vi "生成word报表.vi"(0 "Array输入":refnum<vi>, 1 "产品序号":string, 2 "标注图":T1(plugin-control), 3 "Array输入 2":refnum<vi>, 4 "测试人":string, 5 "部位":string, 6 "ROI左上角X":i32, 7 "ROI左上角Y":i32, 8 "反射图":T1(plugin-control) caption="Original Image", 9 "框号":dbl format="%#_13g") -> (14 "报告生成路径":path)   [LabVIEW 2018]
uses:
  <vilib>/Utility/NIReport.llb/Report Type.ctl
  <vilib>/Utility/NIReport.llb/Append Report Text (str wrap).vi
  <vilib>/addons/_office/word.llb/Word Edit Cell ([dbl]).vi
  <vilib>/addons/_office/word.llb/Word Edit Cell (str).vi
  <vilib>/Utility/NIReport.llb/Append Report Text (num wrap).vi
  <vilib>/Utility/NIReport.llb/NI_report.lvclass
  <vilib>/addons/_office/NI_ReportGenerationToolkit.lvlib
  <vilib>/Utility/NIReport.llb/Word/NI_Word.lvclass
  <vilib>/Utility/NIReport.llb/NI_ReportGenerationCore.lvlib
  <vilib>/addons/_office/word.llb/Word Edit Cell ([str]).vi
panel:
  out "绝对位置Y2":dbl[](array[numeric])
  out "绝对位置X2":dbl[](array[numeric])
  out "绝对位置Y":dbl[](array[numeric])
  out "绝对位置X":dbl[](array[numeric])
  out "分层累计缺陷占比":dbl
  out "分层Z值":dbl[](array[numeric])
  out "缺陷个数 2":i32
  out "分层数据":dbl[][](array[numeric])
  out "弥散累计缺陷占比":dbl
  out "弥散数据":dbl[][](array[numeric])
  out "弥散Z值":dbl[](array[numeric])
  out "缺陷个数":i32
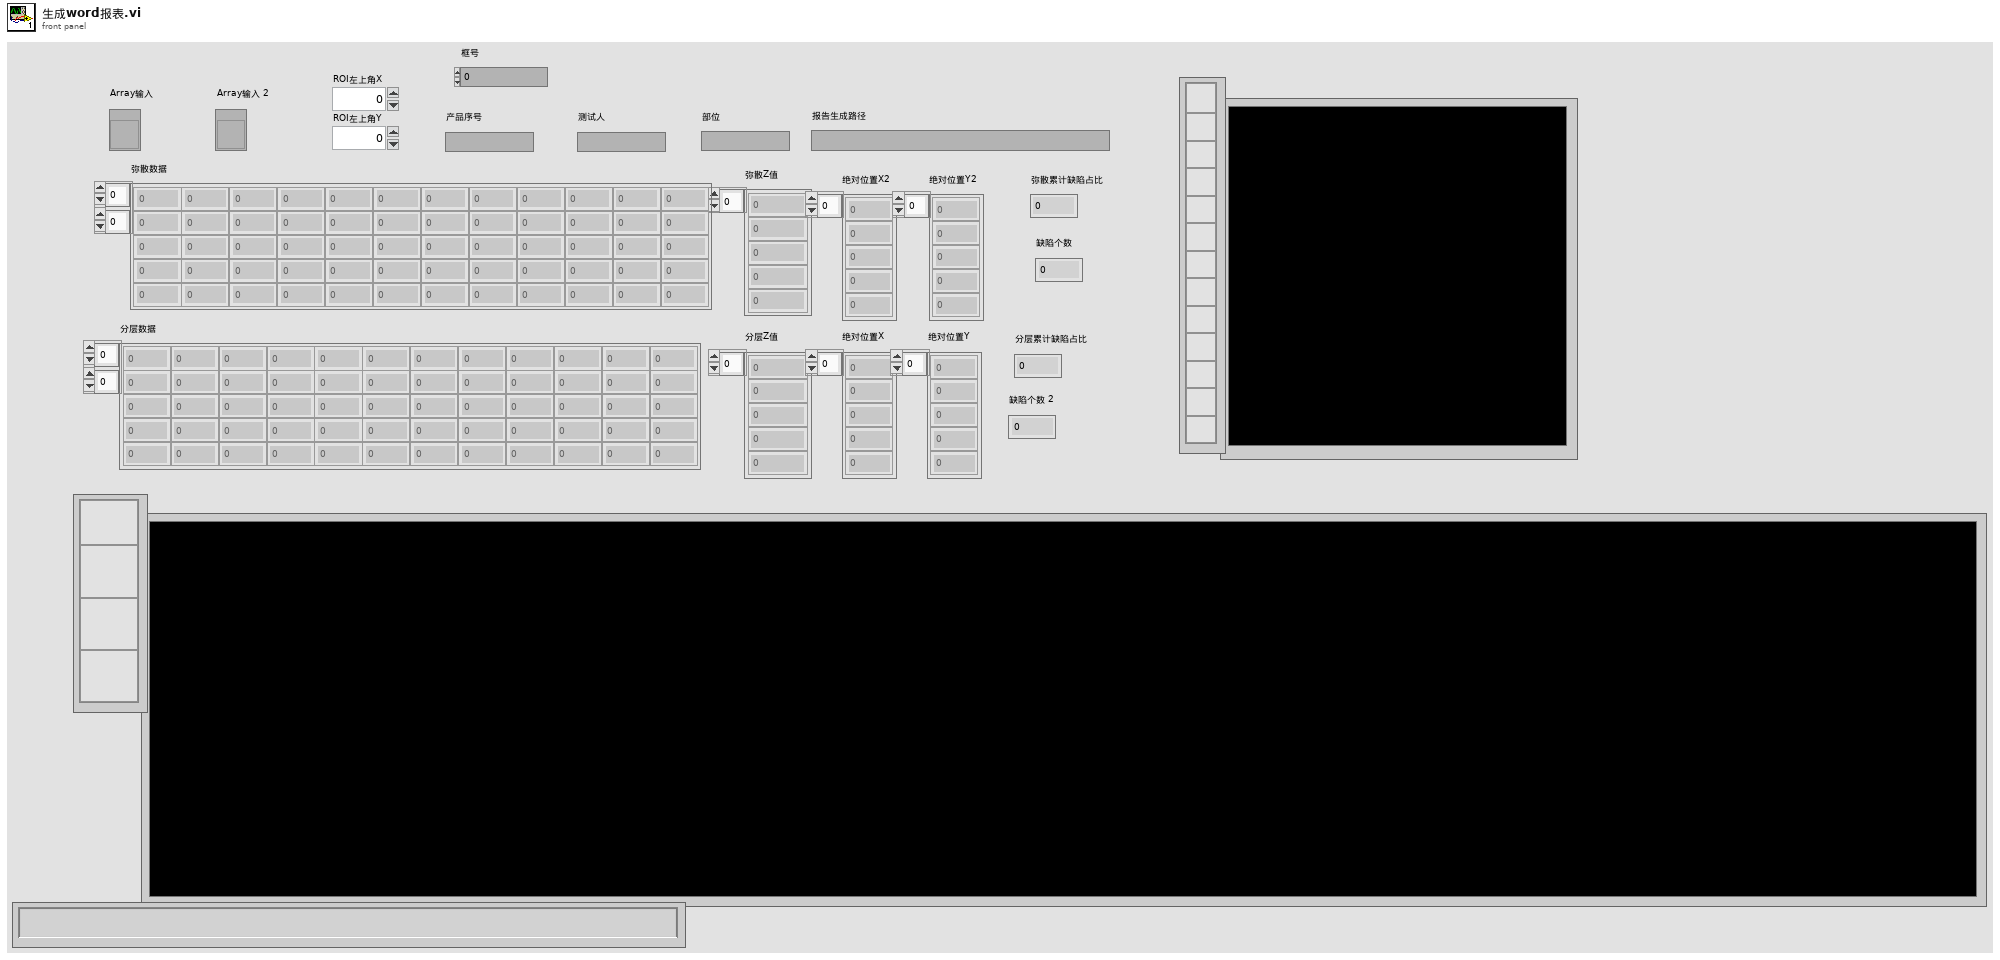
[diagram p1: front panel]
types:
  T1 = typedef "IMAQ Image.ctl" = refnum<image>
  T2 = cluster{"position (Excel)":cluster{"row":i32, "column":i32}, "name (Excel)":string, "bookmark (Word)":string}
  T3 = typedef "NI_ReportGenerationCore.lvlib/Report Type.ctl" = enum16{"HTML", "Word", "Excel"}
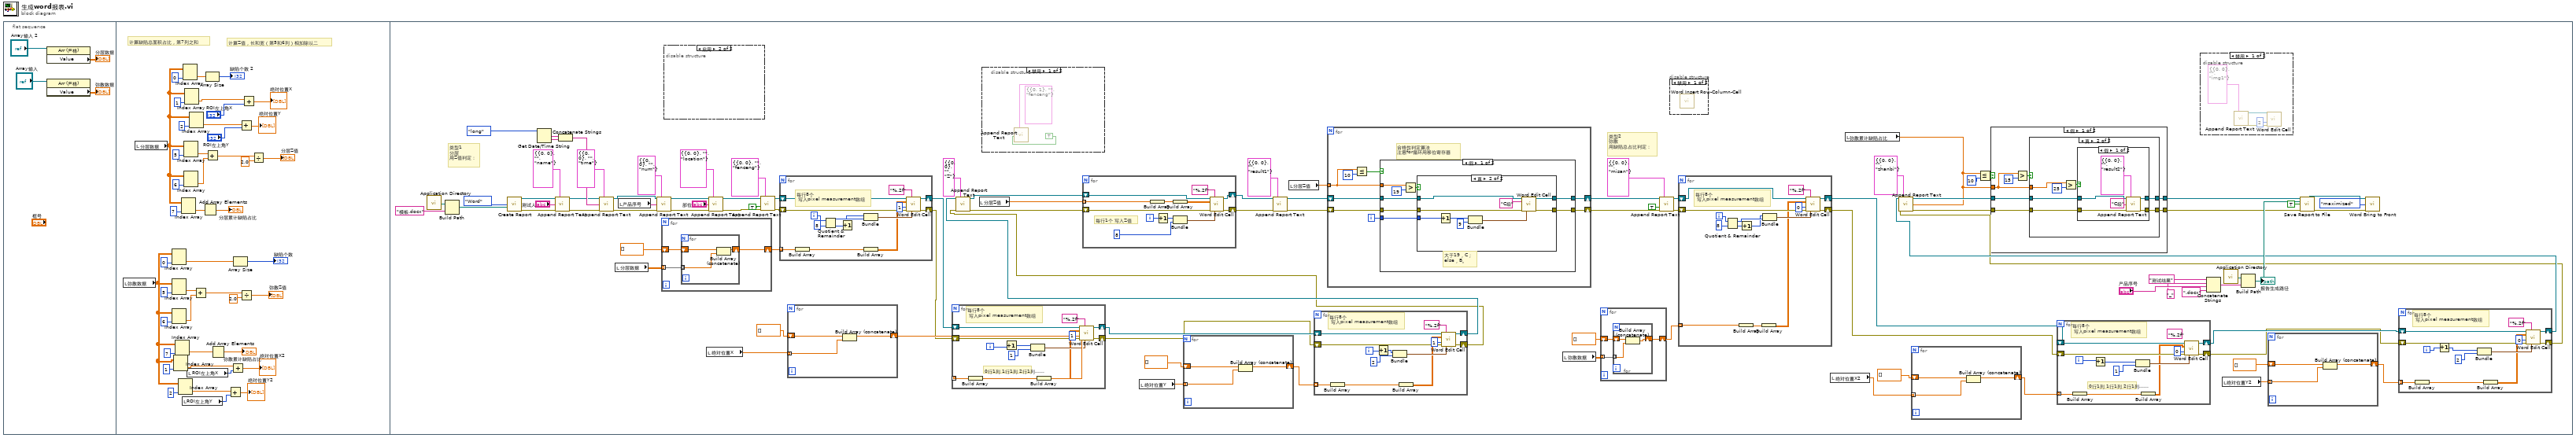
[diagram p0: block diagram]
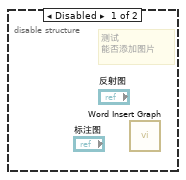
[diagram p5: hidden frame]
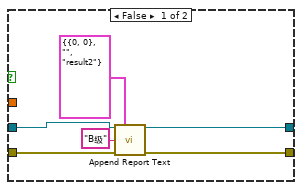
[diagram p6: hidden frame]
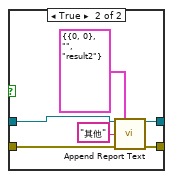
[diagram p7: hidden frame]
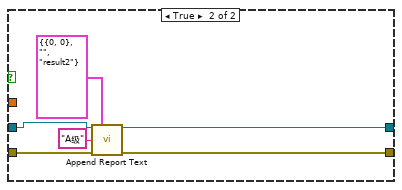
[diagram p8: hidden frame]
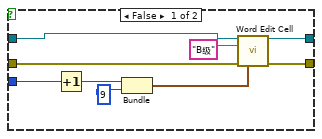
[diagram p9: hidden frame]
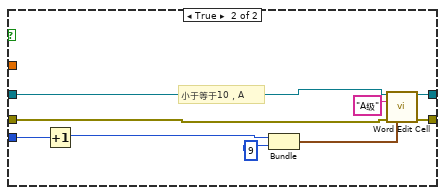
[diagram p10: hidden frame]
diagram:
  n1 = flat-sequence {
    frame #0 {
      n2 = property class="Arr (严格)"(reference="Array输入 2") -> ("Value"=→"分层数据":dbl[][])  [unwired: 1 in, 2 out]
      n3 = property class="Arr (严格)"(reference="Array输入") -> ("Value"=→"弥散数据":dbl[][])  [unwired: 1 in, 2 out]
    }
    frame #1 {
      # "计算缺陷总面积占比，第7列之和"
      # "计算Z值，长和宽（第5和6列）相加除以二"
      n4 = local read "弥散数据"() -> (w7:dbl[][])
      n5 = local read "分层数据"() -> (w20:dbl[][])
      n6 = Index Array(array=w7, index (col)=0 ("禁用的索引 (列)")) -> (element=w46:dbl[])  [unwired: 1 in]
      n7 = Index Array(array=w7, index (col)=5 ("索引")) -> (element=w43:dbl[])  [unwired: 1 in]
      n8 = Index Array(array=w7, index (col)=6 ("索引")) -> (element=w44:dbl[])  [unwired: 1 in]
      n9 = Index Array(array=w7, index (col)=1 ("索引 (列)")) -> (element=w11:dbl[])  [unwired: 1 in]
      n10 = Index Array(array=w7, index (col)=7 ("禁用的索引 (列)")) -> (element=w37:dbl[])  [unwired: 1 in]
      n11 = Index Array(array=w7, index (col)=2 ("索引 (列)")) -> (element=w9:dbl[])  [unwired: 1 in]
      n12 = Index Array(array=w20, index (col)=7 ("禁用的索引 (列)")) -> (element=w24:dbl[])  [unwired: 1 in]
      n13 = local read "ROI左上角Y"() -> (w5:i32)
      n14 = Index Array(array=w20, index (col)=0 ("禁用的索引 (列)")) -> (element=w33:dbl[])  [unwired: 1 in]
      n15 = Index Array(array=w20, index (col)=5 ("索引")) -> (element=w30:dbl[])  [unwired: 1 in]
      n16 = Index Array(array=w20, index (col)=6 ("索引")) -> (element=w31:dbl[])  [unwired: 1 in]
      n17 = Index Array(array=w20, index (col)=1 ("索引 (列)")) -> (element=w19:dbl[])  [unwired: 1 in]
      n18 = local read "ROI左上角X"() -> (w6:i32)
      n19 = Index Array(array=w20, index (col)=2 ("索引 (列)")) -> (element=w16:dbl[])  [unwired: 1 in]
      n20 = Add(x=w43, y=w44) -> (x+y=w45:dbl[])
      n21 = Add Array Elements(numeric array=w24) -> (sum=→"分层累计缺陷占比":dbl)
      n22 = Array Size(array=w33) -> (size(s)=→"缺陷个数 2":i32)
      n23 = Add(x=w30, y=w31) -> (x+y=w32:dbl[])
      n24 = Add Array Elements(numeric array=w37) -> (sum=→"弥散累计缺陷占比":dbl)
      n25 = Add(x=w9, y=w5) -> (x+y=→"绝对位置Y2":dbl[])
      n26 = Add(x=w11, y=w6) -> (x+y=→"绝对位置X2":dbl[])
      n27 = Array Size(array=w46) -> (size(s)=→"缺陷个数":i32)
      n28 = Add(x=w16, y="ROI左上角Y") -> (x+y=→"绝对位置Y":dbl[])
      n29 = Divide(x=w45, y=2.0) -> (x/y=→"弥散Z值":dbl[])
      n30 = Add(x=w19, y="ROI左上角X") -> (x+y=→"绝对位置X":dbl[])
      n31 = Divide(x=w32, y=2.0) -> (x/y=→"分层Z值":dbl[])
    }
    frame #2 {
      # "类型2\n弥散\n用缺陷总占比判定："
      # "类型1\n分层\n用Z值判定："
      n32 = call <vilib>:"Application Directory.vi"() -> ("Application Directory"=w125:path)
      n33 = Build Path(base path=w125, name or relative path="模板.docx") -> (appended path=w124:path)
      n34 = call <vilib>:"Create Report.vi"("report type"=Report_Type."Word" ("Report Type"), "template (empty)"=w124) -> ("report out"=w117:refnum<class "NI_report.lvclass">, "error out"=w114:errorcluster)  [unwired: 12 in]
      n35 = Get Date/Time String(date format (0)=enum16{"short", "long", "abbreviated"}."long" ("日期格式(0)")) -> (date string=w123:string, time string=w121:string)  [unwired: 2 in]
      n36 = call-poly <vilib>:"Append Report Text.vi"("report in"=w117, "MS Office parameters"=T2 {"position (Excel)"={"row"=0, "column"=0}, "name (Excel)"="", "bookmark (Word)"="name"}, "text"="测试人", "error in (no error)"=w114) -> ("report out"=w116:refnum<class "NI_report.lvclass">, "error out"=w115:errorcluster)  [unwired: 8 in, 2 out]
      n37 = Concatenate Strings(w123, w121) -> (w122:string)
      n38 = call-poly <vilib>:"Append Report Text.vi"("report in"=w116, "MS Office parameters"=T2 {"position (Excel)"={"row"=0, "column"=0}, "name (Excel)"="", "bookmark (Word)"="time"}, "text"=w122, "error in (no error)"=w115) -> ("report out"=w120:refnum<class "NI_report.lvclass">, "error out"=w119:errorcluster)  [unwired: 8 in, 2 out]
      n39 = local read "分层数据"() -> (w128:dbl[][])
      n40 = local read "产品序号"() -> (w92:string)
      n41 = call-poly <vilib>:"Append Report Text.vi"("report in"=w120, "MS Office parameters"=T2 {"position (Excel)"={"row"=0, "column"=0}, "name (Excel)"="", "bookmark (Word)"="num"}, "text"=w92, "error in (no error)"=w119) -> ("report out"=w94:refnum<class "NI_report.lvclass">, "error out"=w93:errorcluster)  [unwired: 8 in, 2 out]
      n42 = for {
        tunnel: w128 -> [w328] mode=indexing
        shift-right: [w326] -> w118
        shift-left: dbl[] [] ("元素") -> [w327]
        n43 = for {
          tunnel: w328 -> [w331] mode=indexing
          shift-right: [w329] -> w326
          shift-left: w327 -> [w330]
          n44 = Build Array (concatenate)(w330, w331) -> (w329:dbl[])
        }
      }
      n45 = disable-structure shown="启用" {
        frame Disabled {
          # "测试\n能否添加图片"
          n46 = call <vilib>:"Word Insert Graph.vi"() -> ()  [unwired: 12 in, 4 out]
        }
        frame Enabled {
        }
      }
      n47 = local read "绝对位置X"() -> (w72:dbl[])
      n48 = call-poly <vilib>:"Append Report Text.vi"("report in"=w94, "MS Office parameters"=T2 {"position (Excel)"={"row"=0, "column"=0}, "name (Excel)"="", "bookmark (Word)"="location"}, "text"="部位", "error in (no error)"=w93) -> ("report out"=w96:refnum<class "NI_report.lvclass">, "error out"=w95:errorcluster)  [unwired: 8 in, 2 out]
      n49 = call-poly <vilib>:"Append Report Text.vi"("report in"=w96, "MS Office parameters"=T2 {"position (Excel)"={"row"=0, "column"=0}, "name (Excel)"="", "bookmark (Word)"="fenceng"}, "append on new line? (F)"=TRUE, "error in (no error)"=w95) -> ("report out"=w127:refnum<class "NI_report.lvclass">, "error out"=w126:errorcluster)  [unwired: 8 in, 2 out]
      n50 = for {
        shift-right: [w346] -> w52
        shift-left: w127 -> [w341]
        shift-right: [w345] -> w51
        shift-left: w126 -> [w340]
        tunnel: w118 -> [w334] mode=indexing
        i -> [w342]
        # "每行8个\n 写入pixel measurement数组"
        n51 = Build Array(w334) -> (w336:dbl[])
        n52 = Quotient & Remainder(x=w342, y=8) -> (x-y*floor(x/y)=w339:i32, floor(x/y)=w338:i32)
        n53 = Increment(x=w338) -> (x+1=w337:i32)
        n54 = Bundle(w337, w339) -> (w344:cluster{i32, i32})  [unwired: 1 in]
        n55 = Build Array(w336) -> (w335:dbl[][])
        n56 = call-poly <vilib>:"Word Edit Cell.vi"("report in"=w341, "format string (%.3f)"="%.2f", "value"=w335, "table index (-1)"=i16 1, "error in (no error)"=w340, "start (0, 0)"=w344) -> ("report out"=w346:refnum<class "NI_report.lvclass">, "error out"=w345:errorcluster)  [unwired: 8 in]
      }
      n57 = for {
        tunnel: w72 -> [w194] mode=indexing
        shift-right: [w192] -> w71
        shift-left: dbl[] [] ("元素") -> [w193]
        n58 = Build Array (concatenate)(w193, w194) -> (w192:dbl[])
      }
      n59 = for {
        shift-right: [w207] -> w68
        shift-left: w52 -> [w204]
        shift-right: [w206] -> w67
        shift-left: w51 -> [w203]
        tunnel: w71 -> [w200] mode=indexing
        i -> [w196]
        # "0行1列 1行1列 2行1列......"
        # "每行8个\n 写入pixel measurement数组"
        n60 = Build Array(w200) -> (w202:dbl[])
        n61 = Increment(x=w196) -> (x+1=w195:i32)
        n62 = Bundle(w195, 1) -> (w205:cluster{i32, i32})  [unwired: 1 in]
        n63 = Build Array(w202) -> (w201:dbl[][])
        n64 = call-poly <vilib>:"Word Edit Cell.vi"("report in"=w204, "format string (%.3f)"="%.2f", "value"=w201, "table index (-1)"=i16 1, "error in (no error)"=w203, "start (0, 0)"=w205) -> ("report out"=w207:refnum<class "NI_report.lvclass">, "error out"=w206:errorcluster)  [unwired: 8 in]
      }
      n65 = local read "分层Z值"() -> (w129:dbl[])
      n66 = disable-structure shown="禁用" {
        frame Disabled {
          n67 = call-poly <vilib>:"Append Report Text.vi"("MS Office parameters"=T2 {"position (Excel)"={"row"=0, "column"=1}, "name (Excel)"="", "bookmark (Word)"="fenceng"}, "append on new line? (F)"=TRUE) -> ()  [unwired: 10 in, 4 out]
        }
        frame Enabled {
        }
      }
      n68 = local read "绝对位置Y"() -> (w70:dbl[])
      n69 = for {
        tunnel: w70 -> [w178] mode=indexing
        shift-right: [w176] -> w69
        shift-left: dbl[] [] ("元素") -> [w177]
        n70 = Build Array (concatenate)(w177, w178) -> (w176:dbl[])
      }
      n71 = local read "分层Z值"() -> (w130:dbl[])
      n72 = for {
        shift-right: [w191] -> w66
        shift-left: w68 -> [w188]
        shift-right: [w190] -> w65
        shift-left: w67 -> [w187]
        tunnel: w69 -> [w184] mode=indexing
        i -> [w180]
        # "每行8个\n 写入pixel measurement数组"
        n73 = Build Array(w184) -> (w186:dbl[])
        n74 = Increment(x=w180) -> (x+1=w179:i32)
        n75 = Bundle(w179, 2) -> (w189:cluster{i32, i32})  [unwired: 1 in]
        n76 = Build Array(w186) -> (w185:dbl[][])
        n77 = call-poly <vilib>:"Word Edit Cell.vi"("report in"=w188, "format string (%.3f)"="%.2f", "value"=w185, "table index (-1)"=i16 1, "error in (no error)"=w187, "start (0, 0)"=w189) -> ("report out"=w191:refnum<class "NI_report.lvclass">, "error out"=w190:errorcluster)  [unwired: 8 in]
      }
      n78 = call-poly <vilib>:"Append Report Text.vi"("report in"=w66, "MS Office parameters"=T2 {"position (Excel)"={"row"=0, "column"=0}, "name (Excel)"="", "bookmark (Word)"="Z"}, "error in (no error)"=w65) -> ("report out"=w136:refnum<class "NI_report.lvclass">, "error out"=w135:errorcluster)  [unwired: 9 in, 2 out]
      n79 = for {
        shift-right: [w325] -> w132
        shift-left: w136 -> [w322]
        shift-right: [w324] -> w131
        shift-left: w135 -> [w321]
        tunnel: w129 -> [w317] mode=indexing
        i -> [w315]
        # "每行1个 写入Z值"
        n80 = Build Array(w317) -> (w319:dbl[])
        n81 = Increment(x=w315) -> (x+1=w320:i32)
        n82 = Build Array(w319) -> (w318:dbl[][])
        n83 = Bundle(w320, "y"=8) -> (w323:cluster{i32, "y":i32})  [unwired: 1 in]
        n84 = call-poly <vilib>:"Word Edit Cell.vi"("report in"=w322, "format string (%.3f)"="%.2f", "value"=w318, "error in (no error)"=w321, "start (0, 0)"=w323) -> ("report out"=w325:refnum<class "NI_report.lvclass">, "error out"=w324:errorcluster)  [unwired: 9 in]
      }
      n85 = call-poly <vilib>:"Append Report Text.vi"("report in"=w132, "MS Office parameters"=T2 {"position (Excel)"={"row"=0, "column"=0}, "name (Excel)"="", "bookmark (Word)"="result1"}, "error in (no error)"=w131) -> ("report out"=w133:refnum<class "NI_report.lvclass">, "error out"=w134:errorcluster)  [unwired: 9 in, 2 out]
      n86 = for {
        shift-right: [w272] -> w89
        shift-left: w133 -> [w275]
        shift-right: [w273] -> w88
        shift-left: w134 -> [w274]
        tunnel: w130 -> [w271] mode=indexing
        i -> [w276]
        # "合格性判定算法\n注意for循环用移位寄存器"
        n87 = Less Or Equal?(x=w271, y=10) -> (x <= y?=w277:bool)
        n88 = case shown="假" w277 {
          tunnel: w276 -> [w283 w311]
          tunnel: w275 -> [w282 w310]
          tunnel: w274 -> [w281 w309]
          tunnel: [w279 w308] -> w273
          tunnel: [w280 w307] -> w272
          tunnel: w271 -> [w286 _]
          frame False {
            # "大于19，C；\nelse，B。"
            n89 = Greater?(x=w286, y=19) -> (0:w284:bool)
            n90 = case shown="真" w284 {
              tunnel: w283 -> [w287 w300]
              tunnel: w282 -> [w291 w299]
              tunnel: w281 -> [w290 w298]
              tunnel: [w289 w297] -> w280
              tunnel: [w288 w296] -> w279
              frame False {
                n91 = Increment(x=w287) -> (x+1=w295:i32)
                n92 = Bundle(w295, "y"=9) -> (w294:cluster{i32, "y":i32})  [unwired: 1 in]
                n93 = call-poly <vilib>:"Word Edit Cell.vi"("report in"=w291, "value"="B级", "error in (no error)"=w290, "start (0, 0)"=w294) -> ("report out"=w289:refnum<class "NI_report.lvclass">, "error out"=w288:errorcluster)  [unwired: 10 in]
              }
              frame True {
                n94 = Increment(x=w300) -> (x+1=w304:i32)
                n95 = Bundle(w304, "y"=9) -> (w303:cluster{i32, "y":i32})  [unwired: 1 in]
                n96 = call-poly <vilib>:"Word Edit Cell.vi"("report in"=w299, "value"="C级", "error in (no error)"=w298, "start (0, 0)"=w303) -> ("report out"=w297:refnum<class "NI_report.lvclass">, "error out"=w296:errorcluster)  [unwired: 10 in]
              }
            }
          }
          frame True {
            # "小于等于10，A"
            n97 = Increment(x=w311) -> (x+1=w313:i32)
            n98 = Bundle(w313, "y"=9) -> (w305:cluster{i32, "y":i32})  [unwired: 1 in]
            n99 = call-poly <vilib>:"Word Edit Cell.vi"("report in"=w310, "value"="A级", "error in (no error)"=w309, "start (0, 0)"=w305) -> ("report out"=w307:refnum<class "NI_report.lvclass">, "error out"=w308:errorcluster)  [unwired: 10 in]
          }
        }
      }
      n100 = local read "弥散数据"() -> (w87:dbl[][])
      n101 = for {
        tunnel: w87 -> [w267] mode=indexing
        shift-right: [w265] -> w83
        shift-left: dbl[] [] ("元素") -> [w266]
        n102 = for {
          tunnel: w267 -> [w270] mode=indexing
          shift-right: [w268] -> w265
          shift-left: w266 -> [w269]
          n103 = Build Array (concatenate)(w269, w270) -> (w268:dbl[])
        }
      }
      n104 = call-poly <vilib>:"Append Report Text.vi"("report in"=w89, "MS Office parameters"=T2 {"position (Excel)"={"row"=0, "column"=0}, "name (Excel)"="", "bookmark (Word)"="misan"}, "append on new line? (F)"=TRUE, "error in (no error)"=w88) -> ("report out"=w85:refnum<class "NI_report.lvclass">, "error out"=w84:errorcluster)  [unwired: 8 in, 2 out]
      n105 = disable-structure shown="禁用" {
        frame Disabled {
          n106 = call <vilib>:"Word Insert Row-Column-Cell.vi"() -> ()  [unwired: 14 in, 2 out]
        }
        frame Enabled {
        }
      }
      n107 = for {
        shift-right: [w264] -> w50
        shift-left: w85 -> [w259]
        shift-right: [w263] -> w49
        shift-left: w84 -> [w258]
        tunnel: w83 -> [w252] mode=indexing
        i -> [w260]
        # "每行8个\n 写入pixel measurement数组"
        n108 = Quotient & Remainder(x=w260, y=8) -> (x-y*floor(x/y)=w257:i32, floor(x/y)=w256:i32)
        n109 = Build Array(w252) -> (w254:dbl[])
        n110 = Increment(x=w256) -> (x+1=w255:i32)
        n111 = Build Array(w254) -> (w253:dbl[][])
        n112 = Bundle(w255, w257) -> (w262:cluster{i32, i32})  [unwired: 1 in]
        n113 = call-poly <vilib>:"Word Edit Cell.vi"("report in"=w259, "format string (%.3f)"="%.2f", "value"=w253, "table index (-1)"=i16 0, "error in (no error)"=w258, "start (0, 0)"=w262) -> ("report out"=w264:refnum<class "NI_report.lvclass">, "error out"=w263:errorcluster)  [unwired: 8 in]
      }
      n114 = local read "绝对位置X2"() -> (w54:dbl[])
      n115 = local read "弥散累计缺陷占比"() -> (w77:dbl)
      n116 = for {
        tunnel: w54 -> [w175] mode=indexing
        shift-right: [w173] -> w64
        shift-left: dbl[] [] ("元素") -> [w174]
        n117 = Build Array (concatenate)(w174, w175) -> (w173:dbl[])
      }
      n118 = Less Or Equal?(x=w77, y=10) -> (x <= y?=w78:bool)
      n119 = for {
        shift-right: [w172] -> w61
        shift-left: w50 -> [w169]
        shift-right: [w171] -> w60
        shift-left: w49 -> [w168]
        tunnel: w64 -> [w165] mode=indexing
        i -> [w162]
        (unwired) "%.2f" ("format string (%.3f)")
        # "0行1列 1行1列 2行1列......"
        # "每行8个\n 写入pixel measurement数组"
        n120 = Build Array(w165) -> (w164:dbl[])
        n121 = Increment(x=w162) -> (x+1=w161:i32)
        n122 = Bundle(w161, 1) -> (w170:cluster{i32, i32})  [unwired: 1 in]
        n123 = Build Array(w164) -> (w163:dbl[][])
        n124 = call-poly <vilib>:"Word Edit Cell.vi"("report in"=w169, "value"=w163, "table index (-1)"=i16 0, "error in (no error)"=w168, "start (0, 0)"=w170) -> ("report out"=w172:refnum<class "NI_report.lvclass">, "error out"=w171:errorcluster)  [unwired: 9 in]
      }
      n125 = disable-structure shown="禁用" {
        frame Disabled {
          n126 = call-poly <vilib>:"Append Report Text.vi"("MS Office parameters"=T2 {"position (Excel)"={"row"=0, "column"=0}, "name (Excel)"="", "bookmark (Word)"="img1"}) -> ("report out"=w210:refnum<class "NI_report.lvclass">, "error out"=w209:errorcluster)  [unwired: 11 in, 2 out]
          n127 = call-poly <vilib>:"Word Edit Cell.vi"("report in"=w210, "table index (-1)"=i16 2, "error in (no error)"=w209) -> ()  [unwired: 11 in, 2 out]
        }
        frame Enabled {
        }
      }
      n128 = Concatenate Strings("测试结果" ("字符串"), "_" ("名称或相对路径"), "产品序号", ".docx" ("名称或相对路径")) -> (w140:string)
      n129 = local read "绝对位置Y2"() -> (w62:dbl[])
      n130 = call <vilib>:"Application Directory.vi"() -> ("Application Directory"=w141:path)
      n131 = Build Path(base path=w141, name or relative path=w140) -> (appended path=w142:path)
      "报告生成路径" <- w142
      n132 = for {
        tunnel: w62 -> [w147] mode=indexing
        shift-right: [w145] -> w63
        shift-left: dbl[] [] ("元素") -> [w146]
        n133 = Build Array (concatenate)(w146, w147) -> (w145:dbl[])
      }
      n134 = for {
        shift-right: [w160] -> w59
        shift-left: w61 -> [w157]
        shift-right: [w159] -> w58
        shift-left: w60 -> [w156]
        tunnel: w63 -> [w153] mode=indexing
        i -> [w149]
        # "每行8个\n 写入pixel measurement数组"
        n135 = Build Array(w153) -> (w155:dbl[])
        n136 = Increment(x=w149) -> (x+1=w148:i32)
        n137 = Bundle(w148, 2) -> (w158:cluster{i32, i32})  [unwired: 1 in]
        n138 = Build Array(w155) -> (w154:dbl[][])
        n139 = call-poly <vilib>:"Word Edit Cell.vi"("report in"=w157, "format string (%.3f)"="%.2f", "value"=w154, "table index (-1)"=i16 0, "error in (no error)"=w156, "start (0, 0)"=w158) -> ("report out"=w160:refnum<class "NI_report.lvclass">, "error out"=w159:errorcluster)  [unwired: 8 in]
      }
      n140 = call-poly <vilib>:"Append Report Text.vi"("report in"=w59, "MS Office parameters"=T2 {"position (Excel)"={"row"=0, "column"=0}, "name (Excel)"="", "bookmark (Word)"="zhanbi"}, "text"=w77, "error in (no error)"=w58) -> ("report out"=w81:refnum<class "NI_report.lvclass">, "error out"=w80:errorcluster)  [unwired: 8 in, 2 out]
      n141 = case shown="假" w78 {
        tunnel: w81 -> [w216 w247]
        tunnel: w80 -> [w214 w246]
        tunnel: [w213 w245] -> w73
        tunnel: [w215 w244] -> w74
        tunnel: w77 -> [w212 _]
        frame False {
          n142 = Greater?(x=w212, y=15) -> (0:w217:bool)
          n143 = case shown="真" w217 {
            tunnel: w216 -> [w222 w228]
            tunnel: [w221 w225] -> w215
            tunnel: w214 -> [w220 w227]
            tunnel: [w219 w226] -> w213
            tunnel: w212 -> [_ w230]
            frame False {
              n144 = call-poly <vilib>:"Append Report Text.vi"("report in"=w222, "MS Office parameters"=T2 {"position (Excel)"={"row"=0, "column"=0}, "name (Excel)"="", "bookmark (Word)"="result2"}, "text"="B级", "error in (no error)"=w220) -> ("report out"=w221:refnum<class "NI_report.lvclass">, "error out"=w219:errorcluster)  [unwired: 8 in, 2 out]
            }
            frame True {
              n145 = Greater?(x=w230, y=25) -> (0:w229:bool)
              n146 = case shown="假" w229 {
                tunnel: w228 -> [w235 w241]
                tunnel: w227 -> [w234 w240]
                tunnel: [w233 w239] -> w226
                tunnel: [w232 w238] -> w225
                frame False {
                  n147 = call-poly <vilib>:"Append Report Text.vi"("report in"=w235, "MS Office parameters"=T2 {"position (Excel)"={"row"=0, "column"=0}, "name (Excel)"="", "bookmark (Word)"="result2"}, "text"="C级", "error in (no error)"=w234) -> ("report out"=w232:refnum<class "NI_report.lvclass">, "error out"=w233:errorcluster)  [unwired: 8 in, 2 out]
                }
                frame True {
                  n148 = call-poly <vilib>:"Append Report Text.vi"("report in"=w241, "MS Office parameters"=T2 {"position (Excel)"={"row"=0, "column"=0}, "name (Excel)"="", "bookmark (Word)"="result2"}, "text"="其他", "error in (no error)"=w240) -> ("report out"=w238:refnum<class "NI_report.lvclass">, "error out"=w239:errorcluster)  [unwired: 8 in, 2 out]
                }
              }
            }
          }
        }
        frame True {
          n149 = call-poly <vilib>:"Append Report Text.vi"("report in"=w247, "MS Office parameters"=T2 {"position (Excel)"={"row"=0, "column"=0}, "name (Excel)"="", "bookmark (Word)"="result2"}, "text"="A级", "error in (no error)"=w246) -> ("report out"=w244:refnum<class "NI_report.lvclass">, "error out"=w245:errorcluster)  [unwired: 8 in, 2 out]
        }
      }
      n150 = call-dynamic "Save Report to File.vi"("report in"=w74, "report file path"=w142, "prompt to replace? (F)"=TRUE, "error in (no error)"=w73) -> ("report out"=w139:refnum<class "NI_report.lvclass">, "error out"=w138:errorcluster)  [unwired: 10 in]
      n151 = call <vilib>:"Word Bring to Front.vi"("report in"=w139, "window state (maximized)"=enum16{"maximized", "minimized", "normal"}."maximized", "error in (no error)"=w138) -> ()  [unwired: 11 in, 2 out]
    }
  }
